vi "ConnectToMIDAS.vi"(8 "error in (no error)":errorcluster, 11 "DataPacker in":refnum<class "DataPacker.lvclass">) -> (0 "error out":errorcluster, 2 "Enum":T1, 3 "DataPacker out":refnum<class "DataPacker.lvclass">)   [LabVIEW 2018, in "feGEM DataPacker.lvlib"]
uses:
  feGEM DataPacker.lvlib
  StateMachineTypeDef.ctl
  DataPacker.lvclass
  DataPacker.lvclass/DataPacker.ctl
  DataPacker_ConnectToMIDAS.vi/88b38ab8-c5c0-409b-a7b4-cf79df97607d.vi
  <vilib>/Utility/SystemLogging/Write to System Log.vi
  SendStuff/SayThisOnMIDAS.vi
  DataStructures/GEM_BANK_ARRAY_Add_Data.vi
  DataStructures/GEM_BANK_ARRAY_Flatten.vi
  DataPacker_SendDataToMIDAS.vi
  DataStructures/GEM_BANK_ARRAY.lvclass
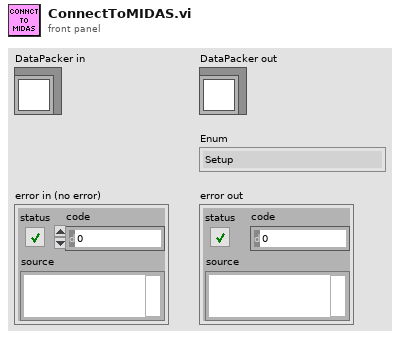
[diagram p1: front panel]
types:
  T1 = typedef "feGEM DataPacker.lvlib/StateMachineTypeDef.ctl" = enum16{"Setup", "Setup SSH", "Connect To Midas", "Get And Set Event Size", "Re-initialise", "Update status", "BundleDataInQueue", "SerializeBundle", "SendData", "Shutdown", "HandleErrorStates", "Wait"}
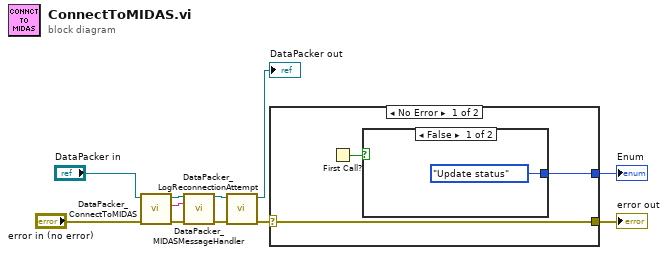
[diagram p0: block diagram]
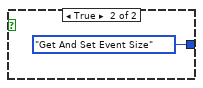
[diagram p2: hidden frame]
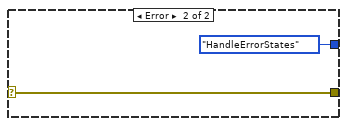
[diagram p3: hidden frame]
diagram:
  n1 = call "DataPacker_ConnectToMIDAS.vi"("error in (no error)"="error in (no error)", "DataPacker in"="DataPacker in") -> ("error out"=w5:errorcluster, "MIDAS Reply"=w4:string, "DataPacker out"=w3:refnum<class "DataPacker.lvclass">)  [unwired: 7 in]
  n2 = call "DataPacker_MIDASMessageHandler.vi"("DataPacker in"=w3, "Message"=w4, "error in (no error)"=w5) -> ("DataPacker out"=w6:refnum<class "DataPacker.lvclass">, "error out"=w7:errorcluster)  [unwired: 11 in]
  n3 = call "DataPacker_LogReconnectionAttempt.vi"("error in (no error)"=w7, "DataPacker in"=w6) -> ("error out"=w9:errorcluster, "DataPacker out"=→"DataPacker out":refnum<class "DataPacker.lvclass">)  [unwired: 8 in]
  n4 = case shown="No Error" w9 {
    selector: w9 -> [w12 w17]
    tunnel: [w14 StateMachineTypeDef."HandleErrorStates" ("Enum")] -> w10
    tunnel: [w12 w17] -> w11
    frame No Error {
      n5 = First Call?() -> (First Call?: T/F=w13:bool)
      n6 = case shown="False" w13 {
        tunnel: [StateMachineTypeDef."Update status" ("Enum") StateMachineTypeDef."Get And Set Event Size" ("Enum")] -> w14
        frame False {
        }
        frame True {
        }
      }
    }
    frame Error {
    }
  }
  "error out" <- w11
  "Enum" <- w10
